vi "getITaskClassPath.vi"() -> (0 "ITaskClassPath":path)   [LabVIEW 2023]
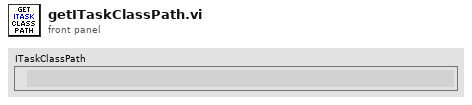
[diagram p1: front panel]
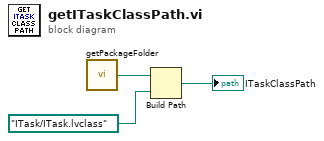
[diagram p0: block diagram]
diagram:
  n1 = call "getPackageFolder.vi"() -> ("packageDirectory"=w2:path)
  n2 = Build Path(base path=w2, name or relative path=path "ITask/ITask.lvclass") -> (appended path=→"ITaskClassPath":path)
